vi "Update Vehicle Out of Position Indicator.vi"(8 "error in (no error)":errorcluster, 10 "Vehicle Out of Pos":bool, 11 "Simulated Wash Display Console in":refnum<class "Simulated Wash Display Console.lvclass">) -> (0 "error out":errorcluster, 3 "Simulated Wash Display Console out":refnum<class "Simulated Wash Display Console.lvclass">)   [LabVIEW 2012, in "Simulated Wash Display Console.lvlib" / "Simulated Wash Display Console.lvclass"]
uses:
  Simulated Wash Display Console.lvclass
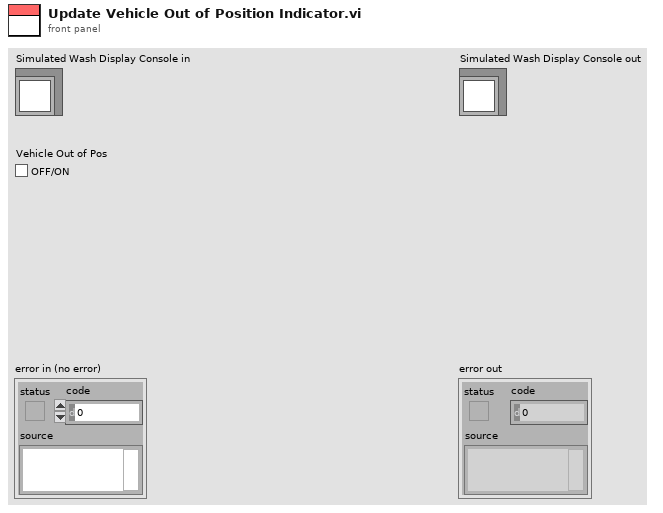
[diagram p1: front panel]
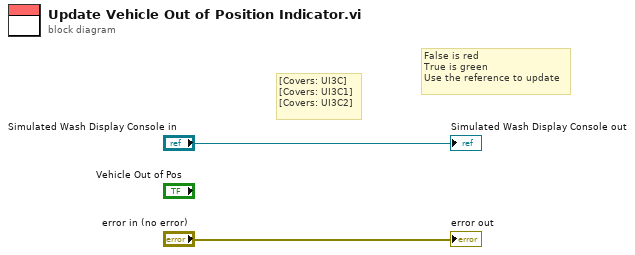
[diagram p0: block diagram]
diagram:
  # "False is red\nTrue is green\nUse the reference to update"
  # "[Covers: UI3C]\n[Covers: UI3C1]\n[Covers: UI3C2]"
  "error out" <- "error in (no error)"
  "Simulated Wash Display Console out" <- "Simulated Wash Display Console in"
